vi "SetListTabletoStr.vi"(4 "Table":string[][](array[string]), 5 "Column Headers[]":string[](array[string])) -> (1 "SetList Table String":string)   [LabVIEW 2013]
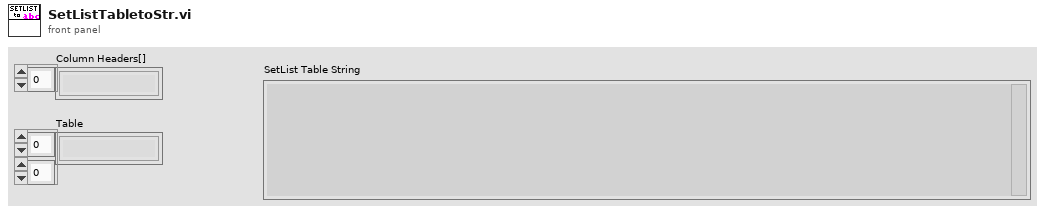
[diagram p1: front panel]
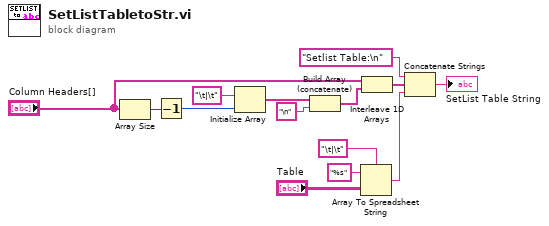
[diagram p0: block diagram]
diagram:
  n1 = Array Size(array="Column Headers[]") -> (size(s)=w11:i32)
  n2 = Decrement(x=w11) -> (x-1=w12:i32)
  n3 = Initialize Array("\t|\t" ("delimiter (Tab)"), w12) -> (w9:string[])
  n4 = Build Array (concatenate)(w9, "\n" ("delimiter (Tab)")) -> (w6:string[])
  n5 = Array To Spreadsheet String(delimiter (Tab)="\t|\t", array="Table", 3:"%s" ("format string")) -> (spreadsheet string=w4:string)
  n6 = Interleave 1D Arrays("Column Headers[]", w6) -> (w5:string[])
  n7 = Concatenate Strings("Setlist Table:\n" ("delimiter (Tab)"), w5, w4) -> (→"SetList Table String":string)
